vi "Generate Packet Log Filename.vi"(8 "error in (no error)":errorcluster) -> (0 "error out":errorcluster, 3 "Filename":string)   [LabVIEW 2013]
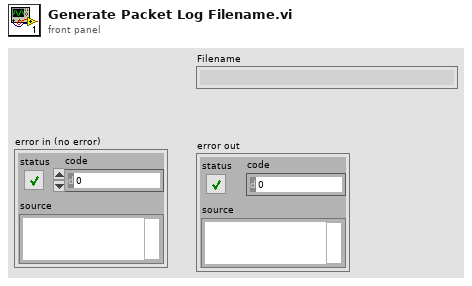
[diagram p1: front panel]
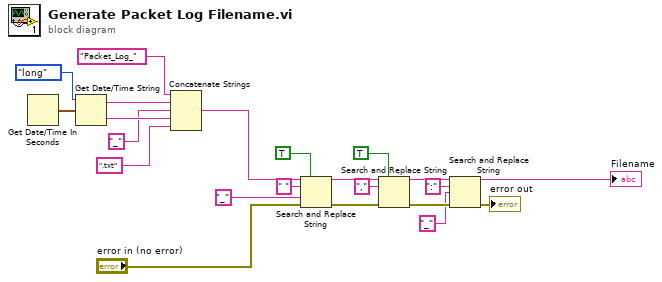
[diagram p0: block diagram]
diagram:
  n1 = Get Date/Time In Seconds() -> (seconds since 1Jan1904=w22:timestamp)
  n2 = Get Date/Time String(date format (0)=enum16{"short", "long", "abbreviated"}."long", seconds (now)=w22) -> (date string=w17:string, time string=w20:string)  [unwired: 1 in]
  n3 = Concatenate Strings("Packet_Log_" ("string"), w17, "_" ("string"), w20, ".txt" ("string")) -> (w19:string)
  n4 = Search and Replace String(replace all?=TRUE ("replace all? (F)"), input string=w19, search string=" ", replace string="_" ("replace string (\"\")"), error in="error in (no error)") -> (result string=w15:string, error out=w8:errorcluster)  [unwired: 3 in, 2 out]
  n5 = Search and Replace String(replace all?=TRUE ("replace all? (F)"), input string=w15, search string=",", error in=w8) -> (result string=w7:string, error out=w6:errorcluster)  [unwired: 4 in, 2 out]
  n6 = Search and Replace String(input string=w7, search string=":", replace string="_" ("replace string (\"\")"), error in=w6) -> (result string=→"Filename":string, error out=→"error out":errorcluster)  [unwired: 4 in, 2 out]
